vi "Selftest.vi"(1 "Swap":bool, 2 "Enc/Dec":enum16{"Encipher", "Decipher"}(ring)) -> (0 "Pass selftest?":bool)   [LabVIEW 2018, in "BlowFish.lvlib"]
uses:
  BlowFish.lvlib
panel:
  out "Text Hex 64bits":string
  out "Pass Hex 4 to 448bits":string
  out "Output Hex 64bits":string
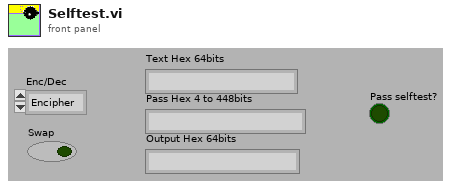
[diagram p1: front panel]
types:
  T1 = cluster{"Password":string, "Plain Text":string, "Cryto Text":string}[]
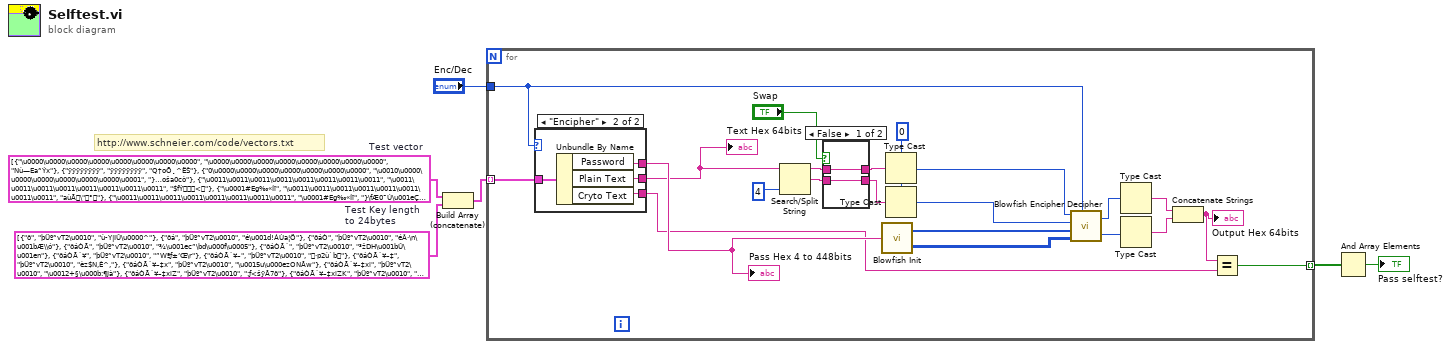
[diagram p0: block diagram]
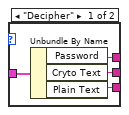
[diagram p2: hidden frame]
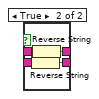
[diagram p3: hidden frame]
diagram:
  w3 = T1 [{"Password"="\u0000\u0000\u0000\u0000\u0000\u0000\u0000\u0000", "Plain Text"="\u0000\u0000\u0000\u0000\u0000\u0000\u0000\u0000", "Cryto Text"="Nù—Ea˜Ýx"}, {"Password"="ÿÿÿÿÿÿÿÿ", "Plain Text"="ÿÿÿÿÿÿÿÿ", "Cryto Text"="Q†oÕ¸^ËŠ"}, {"Password"="0\u0000\u0000\u0000\u0000\u0000\u0000\u0000", "Plain Text"="\u0010\u0000\u0000\u0000\u0000\u0000\u0000\u0001", "Cryto Text"="}…oša0cò"}, {"Password"="\u0011\u0011\u0011\u0011\u0011\u0011\u0011\u0011", "Plain Text"="\u0011\u0011\u0011\u0011\u0011\u0011\u0011\u0011", "Cryto Text"="$fÝ<"}, {"Password"="\u0001#Eg‰«Íï", "Plain Text"="\u0011\u0011\u0011\u0011\u0011\u0011\u0011\u0011", "Cryto Text"="aùÃ\"°"}, {"Password"="\u0011\u0011\u0011\u0011\u0011\u0011\u0011\u0011", "Plain Text"="\u0001#Eg‰«Íï", "Cryto Text"="}\fÆ0¯Ú\u001eÇ"}, {"Password"="\u0000\u0000\u0000\u0000\u0000\u0000\u0000\u0000", "Plain Text"="\u0000\u0000\u0000\u0000\u0000\u0000\u0000\u0000", "Cryto Text"="Nù—Ea˜Ýx"}, {"Password"="þÜº˜vT2\u0010", "Plain Text"="\u0001#Eg‰«Íï", "Cryto Text"="\nÎ«\u000fÆ ¢"}, {"Password"="|¡\u0010EJ\u001anW", "Plain Text"="\u0001¡ÖÐ9wgB", "Cryto Text"="YÆ‚Eë\u0005(+"}, {"Password"="\u00011ÙaÁ7n", "Plain Text"="\\ÕL¨=ïWÚ", "Cryto Text"="±¸Ì\u000b%\u000f\t "}, {"Password"="\u0007¡\u0013>J\u000b&†", "Plain Text"="\u0002HÔ8\u0006öqr", "Cryto Text"="\u00170åw‹ê\u001d¤"}, {"Password"="8IgL&\u00021ž", "Plain Text"="QEKX-ßD\n", "Cryto Text"="¢^xVÏ&Që"}, {"Password"="\u0004¹\u0015ºCþµ¶", "Plain Text"="BýD0YW¢", "Cryto Text"="58±\tÎ\u001a"}, {"Password"="\u0001\u0013¹pý4òÎ", "Plain Text"="\u0005›^\bQÏ\u0014:", "Cryto Text"="HôÐˆL7™\u0018"}, {"Password"="\u0001pñuFµæ", "Plain Text"="\u0007VØàwGaÒ", "Cryto Text"="C!“·‰Qü˜"}, {"Password"="C)­8ãsþ", "Plain Text"="v%\u0014¸)¿Hj", "Cryto Text"="\u0013ðATÖ\u001aå"}, {"Password"="\u0007§\u0013pEÚ*\u0016", "Plain Text"=";Ý\u0011I7(\u0002", "Cryto Text"=".íÚ“ÿÓœy"}, {"Password"="\u0004h‘\u0004Âý;/", "Plain Text"="&•_h5¯`š", "Cryto Text"="Ø‡à9<-¦ã"}, {"Password"="7Ðkµ\u0016ËuF", "Plain Text"="\u0016M^@O'R2", "Cryto Text"="_™ÐO[\u00169i"}, {"Password"="\u001f\b&\r\u001aÂF^", "Plain Text"="k\u0005n\u0018uŸ\\Ê", "Cryto Text"="J\u0005z;$ӗ{"}, {"Password"="X@#d\u001aºav", "Plain Text"="\u0000K诛\t\u0017`b", "Cryto Text"="E 1ÁäúÚŽ"}, {"Password"="\u0002X\u0016\u0016F)°\u0007", "Plain Text"="H\r9\u0000nçbò", "Cryto Text"="uU®9õ›‡½"}, {"Password"="Iy>¼y³%", "Plain Text"="Cu@Èi<ú", "Cryto Text"="SÅ_œ´ŸÀ\u0019"}, {"Password"="O°^\u0015\u0015«s§", "Plain Text"="\u0007-C w\u0007R’", "Cryto Text"="zŽ{ú“~‰£"}, {"Password"="Ié]mL¢)¿", "Plain Text"="\u0002þUw\u0017ñ*", "Cryto Text"="Ïœ]zI†­µ"}, {"Password"="\u0001ƒ\u0010Ü@›&Ö", "Plain Text"="\u001d\\P\u0018÷(Â", "Cryto Text"="Ñ«²eÇx"}, {"Password"="\u001cX\u001c\u0013’Oï", "Plain Text"="0U2(mo)Z", "Cryto Text"="UË7tÑ>ò\u0001"}, {"Password"="\u0001\u0001\u0001\u0001\u0001\u0001\u0001\u0001", "Plain Text"="\u0001#Eg‰«Íï", "Cryto Text"="ú4ìHG²h²"}, {"Password"="\u001f\u001f\u001f\u001f\u000e\u000e\u000e\u000e", "Plain Text"="\u0001#Eg‰«Íï", "Cryto Text"="§yQ\bê<®"}, {"Password"="àþàþñþñþ", "Plain Text"="\u0001#Eg‰«Íï", "Cryto Text"="Ãž\u0007-Ÿ¬c\u001d"}, {"Password"="\u0000\u0000\u0000\u0000\u0000\u0000\u0000\u0000", "Plain Text"="ÿÿÿÿÿÿÿÿ", "Cryto Text"="\u0001I3àÍ¯öä"}, {"Password"="ÿÿÿÿÿÿÿÿ", "Plain Text"="\u0000\u0000\u0000\u0000\u0000\u0000\u0000\u0000", "Cryto Text"="ò\u001ešw·\u001cI¼"}, {"Password"="\u0001#Eg‰«Íï", "Plain Text"="\u0000\u0000\u0000\u0000\u0000\u0000\u0000\u0000", "Cryto Text"="$YFˆWT6š"}, {"Password"="þÜº˜vT2\u0010", "Plain Text"="ÿÿÿÿÿÿÿÿ", "Cryto Text"="k\\Zœ]ž\nZ"}]  # Test vector
  w2 = T1 [{"Password"="ð", "Plain Text"="þÜº˜vT2\u0010", "Cryto Text"="ù­Y|IÛ\u0000^"}, {"Password"="ðá", "Plain Text"="þÜº˜vT2\u0010", "Cryto Text"="é\u001d!ÁÙa¦Ö"}, {"Password"="ðáÒ", "Plain Text"="þÜº˜vT2\u0010", "Cryto Text"="éÂ·\n\u001bÆ\\ó"}, {"Password"="ðáÒÃ", "Plain Text"="þÜº˜vT2\u0010", "Cryto Text"="¾\u001ec”\bd\u000f\u0005"}, {"Password"="ðáÒÃ´", "Plain Text"="þÜº˜vT2\u0010", "Cryto Text"="³žDH\u001bÛ\u001en"}, {"Password"="ðáÒÃ´¥", "Plain Text"="þÜº˜vT2\u0010", "Cryto Text"="”Wªƒ±’Œ\r"}, {"Password"="ðáÒÃ´¥–", "Plain Text"="þÜº˜vT2\u0010", "Cryto Text"="·p2ù`b"}, {"Password"="ðáÒÃ´¥–‡", "Plain Text"="þÜº˜vT2\u0010", "Cryto Text"="èz$N,È^‚"}, {"Password"="ðáÒÃ´¥–‡x", "Plain Text"="þÜº˜vT2\u0010", "Cryto Text"="\u0015u\u000ezONÅw"}, {"Password"="ðáÒÃ´¥–‡xi", "Plain Text"="þÜº˜vT2\u0010", "Cryto Text"="\u0012+§\u000b:¶Jà"}, {"Password"="ðáÒÃ´¥–‡xiZ", "Plain Text"="þÜº˜vT2\u0010", "Cryto Text"=":ƒ<šÿÅ7ö"}, {"Password"="ðáÒÃ´¥–‡xiZK", "Plain Text"="þÜº˜vT2\u0010", "Cryto Text"="”\tÚ‡©\u000fkò"}, {"Password"="ðáÒÃ´¥–‡xiZK<", "Plain Text"="þÜº˜vT2\u0010", "Cryto Text"="ˆO€bP`¸´"}, {"Password"="ðáÒÃ´¥–‡xiZK<-", "Plain Text"="þÜº˜vT2\u0010", "Cryto Text"="\u001f…\u0003\u001c\u0019á\u0019h"}, {"Password"="ðáÒÃ´¥–‡xiZK<-\u001e", "Plain Text"="þÜº˜vT2\u0010", "Cryto Text"="yÙ7:qL£O"}, {"Password"="ðáÒÃ´¥–‡xiZK<-\u001e\u000f", "Plain Text"="þÜº˜vT2\u0010", "Cryto Text"="“\u0014(‡î;á\\"}, {"Password"="ðáÒÃ´¥–‡xiZK<-\u001e\u000f\u0000", "Plain Text"="þÜº˜vT2\u0010", "Cryto Text"="\u0003BžƒŒâÑK"}, {"Password"="ðáÒÃ´¥–‡xiZK<-\u001e\u000f\u0000\u0011", "Plain Text"="þÜº˜vT2\u0010", "Cryto Text"="¤)ž'FŸö{"}, {"Password"="ðáÒÃ´¥–‡xiZK<-\u001e\u000f\u0000\u0011\"", "Plain Text"="þÜº˜vT2\u0010", "Cryto Text"="¯Õ®ÑÁ¼–¨"}, {"Password"="ðáÒÃ´¥–‡xiZK<-\u001e\u000f\u0000\u0011\"3", "Plain Text"="þÜº˜vT2\u0010", "Cryto Text"="\u0010…\u001c\u000e8XÚŸ"}, {"Password"="ðáÒÃ´¥–‡xiZK<-\u001e\u000f\u0000\u0011\"3D", "Plain Text"="þÜº˜vT2\u0010", "Cryto Text"="æõ\u001e×²\u001f"}, {"Password"="ðáÒÃ´¥–‡xiZK<-\u001e\u000f\u0000\u0011\"3DU", "Plain Text"="þÜº˜vT2\u0010", "Cryto Text"="d¦áJý6´o"}, {"Password"="ðáÒÃ´¥–‡xiZK<-\u001e\u000f\u0000\u0011\"3DUf", "Plain Text"="þÜº˜vT2\u0010", "Cryto Text"="€Ç×ÔZTy­"}, {"Password"="ðáÒÃ´¥–‡xiZK<-\u001e\u000f\u0000\u0011\"3DUfw", "Plain Text"="þÜº˜vT2\u0010", "Cryto Text"="\u0005\u0004KbúRÐ€"}]  # Test Key length to 24bytes
  # "http://www.schneier.com/code/vectors.txt"
  n1 = Build Array (concatenate)(w3, w2) -> (w1:T1)
  n2 = for {
    tunnel: [w12] -> w6 mode=indexing
    tunnel: w1 -> [w11] mode=indexing
    tunnel: "Enc/Dec" -> [w7]
    w18 = u32 0
    n3 = case shown="\"Encipher\"" w7 {
      tunnel: w11 -> [w32 w36]
      tunnel: [w31 w35] -> w10
      tunnel: [w30 w34] -> w9
      tunnel: [w29 w33] -> w8
      frame "Decipher" {
        n4 = Unbundle By Name(w32) -> ("Password"=w31:string, "Cryto Text"=w30:string, "Plain Text"=w29:string)
      }
      frame "Encipher" {
        n5 = Unbundle By Name(w36) -> ("Password"=w35:string, "Plain Text"=w34:string, "Cryto Text"=w33:string)
      }
    }
    "Text Hex 64bits" <- w9
    "Pass Hex 4 to 448bits" <- w10
    n6 = Search/Split String(string=w9, offset (0)=4) -> (substring before match=w24:string, match + rest of string=w25:string)  [unwired: 1 in, 1 out]
    n7 = case shown="False" "Swap" {
      tunnel: w24 -> [w38 w42]
      tunnel: w25 -> [w37 w41]
      tunnel: [w38 w40] -> w26
      tunnel: [w37 w39] -> w27
      frame False {
      }
      frame True {
        n8 = Reverse String(1:w41) -> (0:w39:string)
        n9 = Reverse String(1:w42) -> (0:w40:string)
      }
    }
    n10 = call "Blowfish Init.vi"("Key"=w10) -> ("P 18"=w17:u32[], "S 4X256"=w16:u32[][])
    n11 = Type Cast(type=w18, x=w26) -> (*(type *) &x=w15:u32)
    n12 = Type Cast(type=w18, x=w27) -> (*(type *) &x=w14:u32)
    n13 = call "Blowfish Encipher Decipher.vi"("Xl"=w15, "Xr"=w14, "P 18"=w17, "S 4X256"=w16, "Enc/Dec"=w7) -> ("Xl out"=w19:u32, "Xr out"=w20:u32)
    n14 = Type Cast(x=w19) -> (*(type *) &x=w21:string)  [unwired: 1 in]
    n15 = Type Cast(x=w20) -> (*(type *) &x=w22:string)  [unwired: 1 in]
    n16 = Concatenate Strings(w21, w22) -> (w13:string)
    "Output Hex 64bits" <- w13
    n17 = Equal?(x=w13, y=w8) -> (x = y?=w12:bool)
  }
  n18 = And Array Elements(Boolean array=w6) -> (logical AND=→"Pass selftest?":bool)
